vi "KeyenceCVX.File.Read.vi"(7 "log path":path, 8 "error in":errorcluster, 11 "segtings path":path) -> (0 "error out":errorcluster)   [LabVIEW 2016]
uses:
  tools/Tma.lib/nlconfig.llb/fp2ini mode.ctl
  Keyence/LowLevel/Keyence.Global.vi
  KeyenceCVX.Global.vi
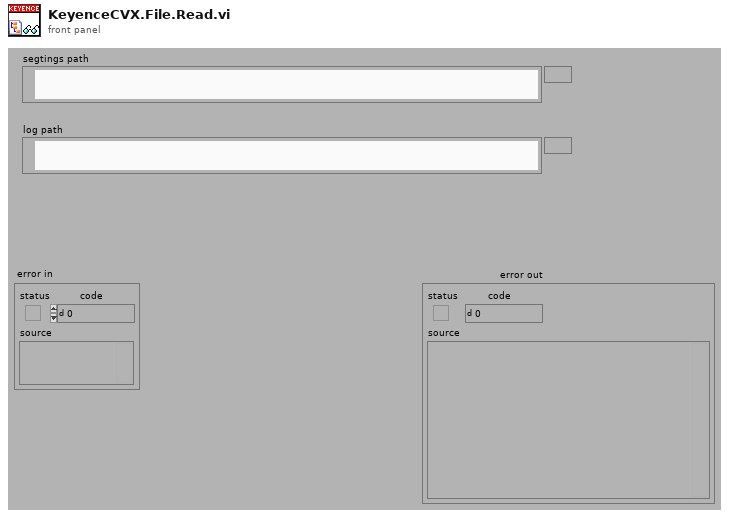
[diagram p1: front panel]
types:
  T1 = typedef "fp2ini mode.ctl" = enum16{"Read Controls", "Write Controls", "Write Indicators", "Read Indicators", "Write all", "Read all"}
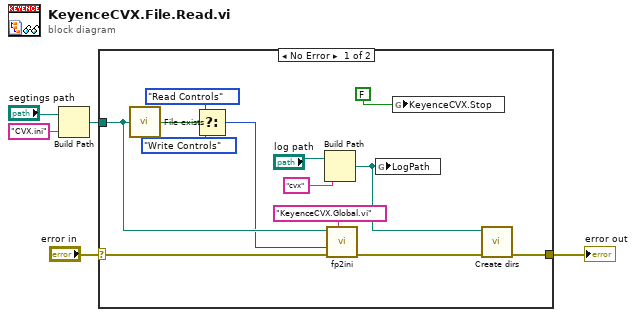
[diagram p0: block diagram]
diagram:
  n1 = Build Path(base path="segtings path", name or relative path="CVX.ini") -> (appended path=w2:path)
  n2 = case shown="No Error" "error in" {
    selector: "error in" -> [w18 w19]
    tunnel: [w8 w19] -> w5
    tunnel: w2 -> [w17 _]
    frame No Error {
      n3 = call "File exists.vi"("file path"=w17) -> ("exists?"=w16:bool)  [unwired: 4 in]
      n4 = Select(t=fp2ini_mode."Read Controls" ("mode"), s=w16, f=fp2ini_mode."Write Controls" ("mode")) -> (s? t:f=w13:T1)
      n5 = Build Path(base path="log path", name or relative path="cvx") -> (appended path=w9:path)
      n6 = call "fp2ini.vi"("vi-name (caller if empty)"="KeyenceCVX.Global.vi", "error in"=w18, "mode"=w13, "ini-file path"=w17) -> ("error out"=w11:errorcluster)  [unwired: 3 in, 4 out]
      n7 = global write "Keyence.Global.vi" "LogPath"(w9) -> ()
      n8 = global write "KeyenceCVX.Global.vi" "KeyenceCVX.Stop"(FALSE ("Keyence.Abort")) -> ()
      n9 = call "Create dirs.vi"("error in (no error)"=w11, "deepest dir"=w9) -> ("error"=w8:errorcluster)  [unwired: 9 in]
    }
    frame Error {
    }
  }
  "error out" <- w5
